vi "Calculate Current.vi"(8 "R1 (Ohms)":dbl=5.0 step=0.1, 11 "Voltage Drop over Load (Volts)":dbl) -> (3 "Current (mA)":dbl format="%#.0f")   [LabVIEW 2015]
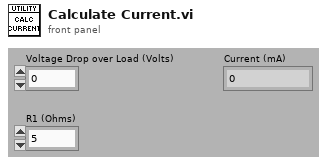
[diagram p1: front panel]
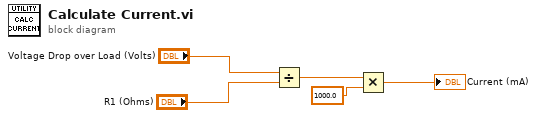
[diagram p0: block diagram]
diagram:
  n1 = Divide(x="Voltage Drop over Load (Volts)", y="R1 (Ohms)") -> (x/y=w2:dbl)
  n2 = Multiply(x=w2, y=1000.0) -> (x*y=→"Current (mA)":dbl)
